vi "Request Header.vi"(8 "error in (no error)":errorcluster, 10 "Header":string, 11 "Processing in":refnum<class "Processing.lvclass">) -> (0 "error out":errorcluster, 1 "Exists":bool, 2 "Value":string, 3 "Processing out":refnum<class "Processing.lvclass">)   [LabVIEW 2020, in "HTTP Server.lvlib" / "Processing.lvclass"]
uses:
  Processing.lvclass
  Processing.lvclass/Processing.ctl
  lv-http-util/HTTP Utils/Request/Request.lvclass
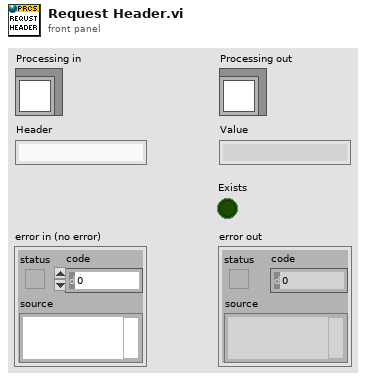
[diagram p1: front panel]
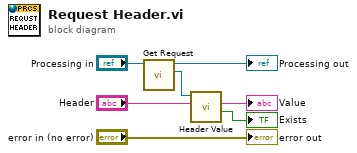
[diagram p0: block diagram]
diagram:
  n1 = call "Get Request.vi"("Processing in"="Processing in") -> ("Request"=w6:refnum<class "Request.lvclass">, "Processing out"=→"Processing out":refnum<class "Processing.lvclass">)  [unwired: 9 in]
  n2 = call "Header Value.vi"("Header"="Header", "Request in"=w6) -> ("Exists"=→"Exists":bool, "Value"=→"Value":string)  [unwired: 6 in, 2 out]
  "error out" <- "error in (no error)"
